vi "Flow.vi"(0 "Flow":dynamicdata(graph), 1 "Cuttoff Pressure":dbl, 5 "Interruption Time":dbl, 7 "SPL":dynamicdata(graph), 9 "File Name In":path, 11 "Error In":errorcluster, 12 "Pressure":dynamicdata(graph)) -> (2 "SPL":dbl format="%0.3f", 3 "Resistance (Out)":dbl, 4 "SGP":dbl, 6 "Interruption Time (Out)":dbl, 8 "PTP":dbl, 10 "File Name":path, 13 "Start Flow":dbl format="%0.3f", 14 "End Flow":dbl format="%0.3f", 15 "Error Out":errorcluster)   [LabVIEW 2020, in "AnalysisSupport.lvlib"]
uses:
  AnalysisSupport.lvlib
  <vilib>/Utility/miscctls.llb/LVCursorListTypeDef.ctl
  <vilib>/Analysis/baseanly.llb/Mean (DBL).vi
  <vilib>/Waveform/WDTOps.llb/WDT Get Waveform Subset DBL.vi
  <vilib>/Analysis/NI_AALBase.lvlib
panel:
  out "Derivative Flow":dynamicdata(graph)
  out "Start Time":dbl format="%#.3g"
  in  "Resistance":dbl step=5.0
  out "Subset":dynamicdata(graph)
  out "Flow":dynamicdata(graph)
  in  "Mark Flow":bool
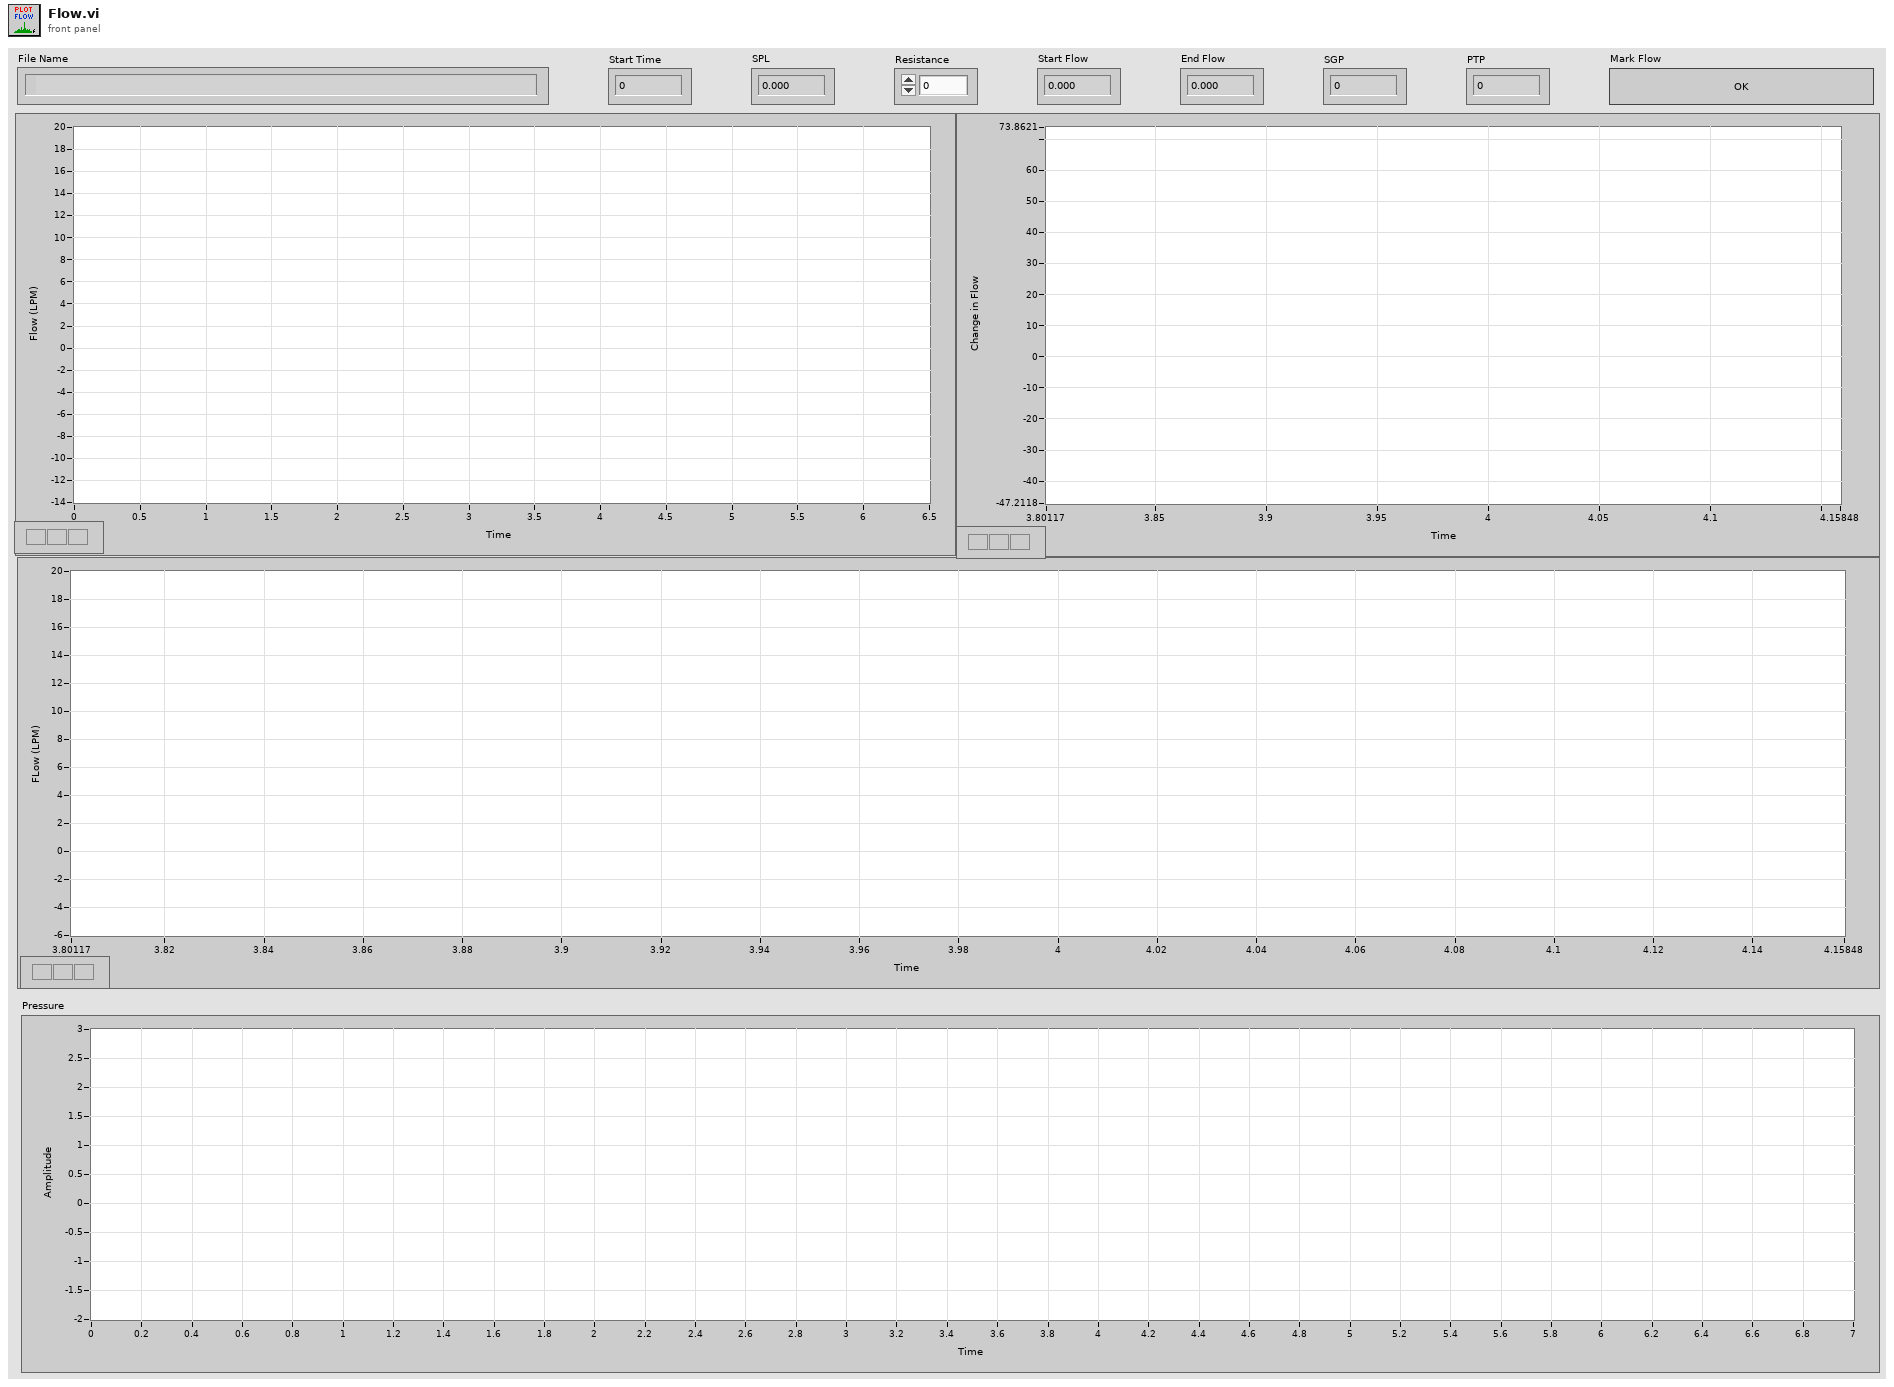
[diagram p1: front panel]
types:
  T1 = typedef "LVCursorListTypeDef.ctl" = cluster{"Name":string, "Color":u32, "Style":u8, "Point Style":u8, "Name Visible":bool, "Allow Drag":bool, "Cursor Mode":u32, "Plot":i32, "Index":i32, "Position":cluster{"X":dbl, "Y":dbl}, "X Scale":u32, "Y Scale":u32, "Watch Plots":i32[], "Watch All Plots":bool, "Plot Area":i32, "Label Offset":cluster{"X":dbl, "Y":dbl}}[]
  T2 = cluster{"Cursor List[0]":cluster{"Name":string, "Color":u32, "Style":u8, "Point Style":u8, "Name Visible":bool, "Allow Drag":bool, "Cursor Mode":u32, "Plot":i32, "Index":i32, "Position":cluster{"X":dbl, "Y":dbl}, "X Scale":u32, "Y Scale":u32, "Watch Plots":i32[], "Watch All Plots":bool, "Plot Area":i32, "Label Offset":cluster{"X":dbl, "Y":dbl}}, "Cursor List[1]":cluster{"Name":string, "Color":u32, "Style":u8, "Point Style":u8, "Name Visible":bool, "Allow Drag":bool, "Cursor Mode":u32, "Plot":i32, "Index":i32, "Position":cluster{"X":dbl, "Y":dbl}, "X Scale":u32, "Y Scale":u32, "Watch Plots":i32[], "Watch All Plots":bool, "Plot Area":i32, "Label Offset":cluster{"X":dbl, "Y":dbl}}, "Cursor List[2]":cluster{"Name":string, "Color":u32, "Style":u8, "Point Style":u8, "Name Visible":bool, "Allow Drag":bool, "Cursor Mode":u32, "Plot":i32, "Index":i32, "Position":cluster{"X":dbl, "Y":dbl}, "X Scale":u32, "Y Scale":u32, "Watch Plots":i32[], "Watch All Plots":bool, "Plot Area":i32, "Label Offset":cluster{"X":dbl, "Y":dbl}}, "Cursor List[3]":cluster{"Name":string, "Color":u32, "Style":u8, "Point Style":u8, "Name Visible":bool, "Allow Drag":bool, "Cursor Mode":u32, "Plot":i32, "Index":i32, "Position":cluster{"X":dbl, "Y":dbl}, "X Scale":u32, "Y Scale":u32, "Watch Plots":i32[], "Watch All Plots":bool, "Plot Area":i32, "Label Offset":cluster{"X":dbl, "Y":dbl}}, "Cursor List[4]":cluster{"Name":string, "Color":u32, "Style":u8, "Point Style":u8, "Name Visible":bool, "Allow Drag":bool, "Cursor Mode":u32, "Plot":i32, "Index":i32, "Position":cluster{"X":dbl, "Y":dbl}, "X Scale":u32, "Y Scale":u32, "Watch Plots":i32[], "Watch All Plots":bool, "Plot Area":i32, "Label Offset":cluster{"X":dbl, "Y":dbl}}, "Cursor List[5]":cluster{"Name":string, "Color":u32, "Style":u8, "Point Style":u8, "Name Visible":bool, "Allow Drag":bool, "Cursor Mode":u32, "Plot":i32, "Index":i32, "Position":cluster{"X":dbl, "Y":dbl}, "X Scale":u32, "Y Scale":u32, "Watch Plots":i32[], "Watch All Plots":bool, "Plot Area":i32, "Label Offset":cluster{"X":dbl, "Y":dbl}}, "Cursor List[6]":cluster{"Name":string, "Color":u32, "Style":u8, "Point Style":u8, "Name Visible":bool, "Allow Drag":bool, "Cursor Mode":u32, "Plot":i32, "Index":i32, "Position":cluster{"X":dbl, "Y":dbl}, "X Scale":u32, "Y Scale":u32, "Watch Plots":i32[], "Watch All Plots":bool, "Plot Area":i32, "Label Offset":cluster{"X":dbl, "Y":dbl}}, "Cursor List[7]":cluster{"Name":string, "Color":u32, "Style":u8, "Point Style":u8, "Name Visible":bool, "Allow Drag":bool, "Cursor Mode":u32, "Plot":i32, "Index":i32, "Position":cluster{"X":dbl, "Y":dbl}, "X Scale":u32, "Y Scale":u32, "Watch Plots":i32[], "Watch All Plots":bool, "Plot Area":i32, "Label Offset":cluster{"X":dbl, "Y":dbl}}, "Cursor List[8]":cluster{"Name":string, "Color":u32, "Style":u8, "Point Style":u8, "Name Visible":bool, "Allow Drag":bool, "Cursor Mode":u32, "Plot":i32, "Index":i32, "Position":cluster{"X":dbl, "Y":dbl}, "X Scale":u32, "Y Scale":u32, "Watch Plots":i32[], "Watch All Plots":bool, "Plot Area":i32, "Label Offset":cluster{"X":dbl, "Y":dbl}}}
  T3 = cluster{"Name":string, "Color":u32, "Style":u8, "Point Style":u8, "Name Visible":bool, "Allow Drag":bool, "Cursor Mode":u32, "Plot":i32, "Index":i32, "Position":cluster{"X":dbl, "Y":dbl}, "X Scale":u32, "Y Scale":u32, "Watch Plots":i32[], "Watch All Plots":bool, "Plot Area":i32, "Label Offset":cluster{"X":dbl, "Y":dbl}}[]
  T4 = cluster{"CrsrList[0]":cluster{"Name":string, "Color":u32, "Style":u8, "Point Style":u8, "Name Visible":bool, "Allow Drag":bool, "Cursor Mode":u32, "Plot":i32, "Index":i32, "Position":cluster{"X":dbl, "Y":dbl}, "X Scale":u32, "Y Scale":u32, "Watch Plots":i32[], "Watch All Plots":bool, "Plot Area":i32, "Label Offset":cluster{"X":dbl, "Y":dbl}}, "CrsrList[1]":cluster{"Name":string, "Color":u32, "Style":u8, "Point Style":u8, "Name Visible":bool, "Allow Drag":bool, "Cursor Mode":u32, "Plot":i32, "Index":i32, "Position":cluster{"X":dbl, "Y":dbl}, "X Scale":u32, "Y Scale":u32, "Watch Plots":i32[], "Watch All Plots":bool, "Plot Area":i32, "Label Offset":cluster{"X":dbl, "Y":dbl}}, "CrsrList[2]":cluster{"Name":string, "Color":u32, "Style":u8, "Point Style":u8, "Name Visible":bool, "Allow Drag":bool, "Cursor Mode":u32, "Plot":i32, "Index":i32, "Position":cluster{"X":dbl, "Y":dbl}, "X Scale":u32, "Y Scale":u32, "Watch Plots":i32[], "Watch All Plots":bool, "Plot Area":i32, "Label Offset":cluster{"X":dbl, "Y":dbl}}, "CrsrList[3]":cluster{"Name":string, "Color":u32, "Style":u8, "Point Style":u8, "Name Visible":bool, "Allow Drag":bool, "Cursor Mode":u32, "Plot":i32, "Index":i32, "Position":cluster{"X":dbl, "Y":dbl}, "X Scale":u32, "Y Scale":u32, "Watch Plots":i32[], "Watch All Plots":bool, "Plot Area":i32, "Label Offset":cluster{"X":dbl, "Y":dbl}}, "CrsrList[4]":cluster{"Name":string, "Color":u32, "Style":u8, "Point Style":u8, "Name Visible":bool, "Allow Drag":bool, "Cursor Mode":u32, "Plot":i32, "Index":i32, "Position":cluster{"X":dbl, "Y":dbl}, "X Scale":u32, "Y Scale":u32, "Watch Plots":i32[], "Watch All Plots":bool, "Plot Area":i32, "Label Offset":cluster{"X":dbl, "Y":dbl}}, "CrsrList[5]":cluster{"Name":string, "Color":u32, "Style":u8, "Point Style":u8, "Name Visible":bool, "Allow Drag":bool, "Cursor Mode":u32, "Plot":i32, "Index":i32, "Position":cluster{"X":dbl, "Y":dbl}, "X Scale":u32, "Y Scale":u32, "Watch Plots":i32[], "Watch All Plots":bool, "Plot Area":i32, "Label Offset":cluster{"X":dbl, "Y":dbl}}, "CrsrList[6]":cluster{"Name":string, "Color":u32, "Style":u8, "Point Style":u8, "Name Visible":bool, "Allow Drag":bool, "Cursor Mode":u32, "Plot":i32, "Index":i32, "Position":cluster{"X":dbl, "Y":dbl}, "X Scale":u32, "Y Scale":u32, "Watch Plots":i32[], "Watch All Plots":bool, "Plot Area":i32, "Label Offset":cluster{"X":dbl, "Y":dbl}}, "CrsrList[7]":cluster{"Name":string, "Color":u32, "Style":u8, "Point Style":u8, "Name Visible":bool, "Allow Drag":bool, "Cursor Mode":u32, "Plot":i32, "Index":i32, "Position":cluster{"X":dbl, "Y":dbl}, "X Scale":u32, "Y Scale":u32, "Watch Plots":i32[], "Watch All Plots":bool, "Plot Area":i32, "Label Offset":cluster{"X":dbl, "Y":dbl}}, "CrsrList[8]":cluster{"Name":string, "Color":u32, "Style":u8, "Point Style":u8, "Name Visible":bool, "Allow Drag":bool, "Cursor Mode":u32, "Plot":i32, "Index":i32, "Position":cluster{"X":dbl, "Y":dbl}, "X Scale":u32, "Y Scale":u32, "Watch Plots":i32[], "Watch All Plots":bool, "Plot Area":i32, "Label Offset":cluster{"X":dbl, "Y":dbl}}}
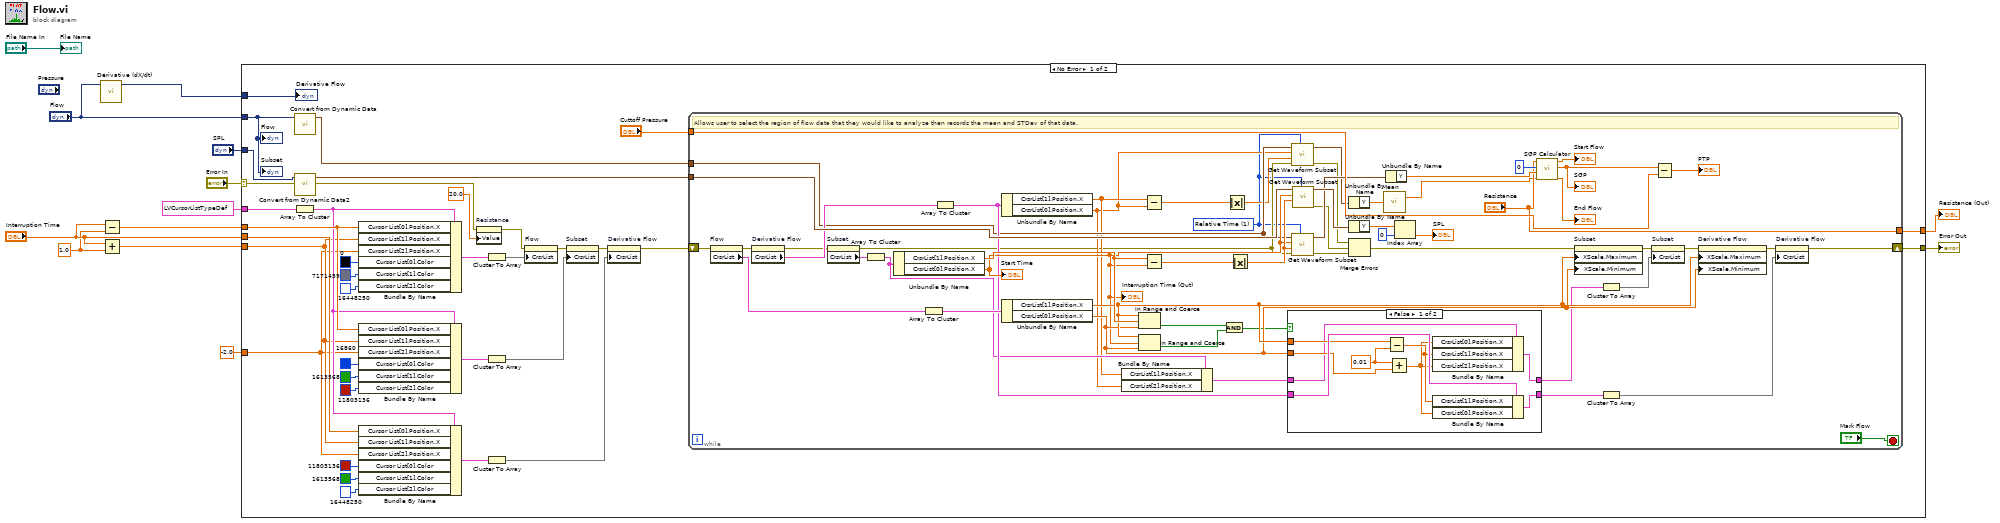
[diagram p0: block diagram]
diagram:
  w3 = 1.0 ("y")
  n1 = call "Derivative (dX/dt)"("Signals"="Flow") -> ("Result"=w5:dynamicdata)  [unwired: 5 in, 1 out]
  n2 = Subtract(x="Interruption Time", y=w3) -> (x-y=w7:dbl)
  n3 = Add(x="Interruption Time", y=w3) -> (x+y=w4:dbl)
  n4 = case shown="No Error" "Error In" {
    selector: "Error In" -> [w29 w116]
    tunnel: "Flow" -> [w47 _]
    tunnel: [w48 w116] -> w11
    tunnel: "Interruption Time" -> [w44 _]
    tunnel: T1 [{"Name"="Left", "Color"=9843450, "Style"=2, "Point Style"=1, "Name Visible"=FALSE, "Allow Drag"=TRUE, "Cursor Mode"=0, "Plot"=0, "Index"=0, "Position"={"X"=3.0, "Y"=0.0}, "X Scale"=0, "Y Scale"=0, "Watch Plots"=[], "Watch All Plots"=FALSE, "Plot Area"=0, "Label Offset"={"X"=0.0, "Y"=0.0}}, {"Name"="Right", "Color"=681210, "Style"=2, "Point Style"=1, "Name Visible"=FALSE, "Allow Drag"=TRUE, "Cursor Mode"=0, "Plot"=0, "Index"=0, "Position"={"X"=3.5, "Y"=0.0}, "X Scale"=0, "Y Scale"=0, "Watch Plots"=[], "Watch All Plots"=FALSE, "Plot Area"=0, "Label Offset"={"X"=0.0, "Y"=0.0}}, {"Name"="Middle", "Color"=4617539, "Style"=2, "Point Style"=1, "Name Visible"=FALSE, "Allow Drag"=TRUE, "Cursor Mode"=0, "Plot"=0, "Index"=0, "Position"={"X"=0.0, "Y"=0.0}, "X Scale"=0, "Y Scale"=0, "Watch Plots"=[], "Watch All Plots"=FALSE, "Plot Area"=0, "Label Offset"={"X"=0.0, "Y"=0.0}}] ("Cursor List") -> [w45 _]
    tunnel: [w42 _] -> w9
    tunnel: w4 -> [w24 _]
    tunnel: w7 -> [w26 _]
    tunnel: "SPL" -> [w37 _]
    tunnel: w5 -> [w34 _]
    tunnel: -2.0 -> [w23 _]
    frame No Error {
      n5 = call "Convert from Dynamic Data"("Dynamic Data Type"=w47) -> ("Waveform"=w46:waveform(dbl))  [unwired: 3 in]
      n6 = call "Convert from Dynamic Data2"("Dynamic Data Type"=w37) -> ("Waveform"=w36:waveform(dbl))  [unwired: 3 in]
      n7 = Array To Cluster(array=w45) -> (cluster=w25:T2)
      n8 = Bundle By Name(cluster=w25, "Cursor List[0].Position.X"=w26, "Cursor List[1].Position.X"=w24, "Cursor List[2].Position.X"=w23, "Cursor List[0].Color"=u32 0, "Cursor List[1].Color"=u32 7171459, "Cursor List[2].Color"=u32 16448250) -> (w40:T2)
      n9 = Bundle By Name(cluster=w25, "Cursor List[0].Position.X"=w26, "Cursor List[1].Position.X"=w24, "Cursor List[2].Position.X"=w23, "Cursor List[0].Color"=u32 16860, "Cursor List[1].Color"=u32 1613568, "Cursor List[2].Color"=u32 11803136) -> (w28:T2)
      n10 = Bundle By Name(cluster=w25, "Cursor List[0].Position.X"=w44, "Cursor List[1].Position.X"=w24, "Cursor List[2].Position.X"=w23, "Cursor List[0].Color"=u32 11803136, "Cursor List[1].Color"=u32 1613568, "Cursor List[2].Color"=u32 16448250) -> (w43:T2)
      n11 = property on="Resistance" class="DigNum (strict)"(error in=w29, "Value"=20.0 ("Resistance")) -> (error out=w30:errorcluster)  [unwired: 1 in, 1 out]
      n12 = Cluster To Array(cluster=w40) -> (array=w39:T3)
      n13 = Cluster To Array(cluster=w28) -> (array=w27:T3)
      n14 = Cluster To Array(cluster=w43) -> (array=w31:T3)
      n15 = property on="Flow" class="WFGraph (strict)"(error in=w30, "CrsrList"=w39) -> (error out=w41:errorcluster)  [unwired: 1 in, 1 out]
      n16 = property on="Subset" class="WFGraph (strict)"(error in=w41, "CrsrList"=w27) -> (error out=w33:errorcluster)  [unwired: 1 in, 1 out]
      n17 = property on="Derivative Flow" class="WFGraph (strict)"(error in=w33, "CrsrList"=w31) -> (error out=w32:errorcluster)  [unwired: 1 in, 1 out]
      n18 = while {
        shift-right: [w71] -> w48
        shift-left: w32 -> [w77]
        tunnel: w46 -> [w68]
        tunnel: ["Resistance"] -> w42
        tunnel: w36 -> [w97]
        tunnel: "Cuttoff Pressure" -> [w96]
        stop <- "Mark Flow" stop-if-true
        w49 = u16 1 items=["Samples", "Relative Time"] ("start/duration format")
        # "Allows user to select the region of flow data that they would like to analyze then records the mean and STDev of that data."
        n19 = property on="Flow" class="WFGraph (strict)"(error in=w77) -> (error out=w55:errorcluster, "CrsrList"=w102:T1)  [unwired: 1 in, 1 out]
        n20 = property on="Derivative Flow" class="WFGraph (strict)"(error in=w55) -> (error out=w54:errorcluster, "CrsrList"=w95:T1)  [unwired: 1 in, 1 out]
        n21 = property on="Subset" class="WFGraph (strict)"(error in=w54) -> (error out=w52:errorcluster, "CrsrList"=w101:T1)  [unwired: 1 in, 1 out]
        n22 = Array To Cluster(array=w101) -> (cluster=w67:T4)
        n23 = Unbundle By Name(w67) -> ("CrsrList[1].Position.X"=w100:dbl, "CrsrList[0].Position.X"=w78:dbl)
        "Interruption Time (Out)" <- w78
        "Start Time" <- w78
        n24 = Array To Cluster(array=w102) -> (cluster=w103:T4)
        n25 = Array To Cluster(array=w95) -> (cluster=w70:T4)
        n26 = Unbundle By Name(w70) -> ("CrsrList[1].Position.X"=w59:dbl, "CrsrList[0].Position.X"=w58:dbl)
        n27 = Unbundle By Name(w103) -> ("CrsrList[1].Position.X"=w99:dbl, "CrsrList[0].Position.X"=w98:dbl)
        n28 = Bundle By Name(cluster=w67, "CrsrList[1].Position.X"=w59, "CrsrList[2].Position.X"=w58) -> (w66:T4)
        n29 = In Range and Coerce(upper limit=w99, x=w100, lower limit=w98) -> (In Range?=w93:bool)  [unwired: 1 out]
        n30 = In Range and Coerce(upper limit=w99, x=w78, lower limit=w98) -> (In Range?=w92:bool)  [unwired: 1 out]
        n31 = Subtract(x=w59, y=w58) -> (x-y=w60:dbl)
        n32 = Subtract(x=w100, y=w78) -> (x-y=w90:dbl)
        n33 = And(x=w93, y=w92) -> (x .and. y?=w91:bool)
        n34 = Absolute Value(x=w60) -> (abs(x)=w61:dbl)
        n35 = Absolute Value(x=w90) -> (abs(x)=w86:dbl)
        n36 = case shown="False" w91 {
          tunnel: w70 -> [w113 w115]
          tunnel: [w112 w115] -> w94
          tunnel: w99 -> [w111 _]
          tunnel: w98 -> [w110 _]
          tunnel: w66 -> [w109 w114]
          tunnel: [w108 w114] -> w74
          frame False {
            w107 = 0.01 ("y")
            # "Right Cursor"
            n37 = Subtract(x=w111, y=w107) -> (x-y=w106:dbl)
            n38 = Add(x=w107, y=w110) -> (x+y=w105:dbl)
            n39 = Bundle By Name(cluster=w109, "CrsrList[0].Position.X"=w105, "CrsrList[1].Position.X"=w106, "CrsrList[2].Position.X"=w105) -> (w108:T4)
            n40 = Bundle By Name(cluster=w113, "CrsrList[1].Position.X"=w106, "CrsrList[0].Position.X"=w105) -> (w112:T4)
          }
          frame True {
            # "Right Cursor"
          }
        }
        n41 = call-poly <vilib>:"Get Waveform Subset.vi"("start/duration format"=w49, "error in (no error)"=w52, "duration"=w61, "start samples/time"=w58, "waveform in"=w68) -> ("error out"=w57:errorcluster, "waveform out"=w64:waveform(dbl))  [unwired: 1 in, 2 out]
        n42 = call-poly <vilib>:"Get Waveform Subset.vi"("start/duration format"=w49, "error in (no error)"=w52, "duration"=w86, "start samples/time"=w78, "waveform in"=w68) -> ("error out"=w50:errorcluster, "waveform out"=w69:waveform(dbl))  [unwired: 1 in, 2 out]
        n43 = call-poly <vilib>:"Get Waveform Subset.vi"("start/duration format"=w49, "duration"=w86, "start samples/time"=w78, "waveform in"=w97) -> ("error out"=w56:errorcluster, "waveform out"=w87:waveform(dbl))  [unwired: 2 in, 2 out]
        n44 = Unbundle By Name(w64) -> ("Y"=w63:dbl[])
        n45 = Unbundle By Name(w87) -> ("Y"=w85:dbl[])
        n46 = Merge Errors(w57, w56, w50) -> (w51:errorcluster)
        n47 = call-poly <vilib>:"Mean.vi"("X"=w63) -> ("mean"=w62:dbl)  [unwired: 1 out]
        n48 = Unbundle By Name(w69) -> ("Y"=w88:dbl[])
        n49 = Index Array(array=w85, index=0 ("Start Index")) -> (element=→"SPL":dbl)
        n50 = call "SGP Calculator.vi"("End Flow"=w62, "Flow Array"=w88, "Start Index"=0, "Resistance"="Resistance") -> ("End Flow Out"=→"End Flow":dbl, "SGP"=w80:dbl, "Start Flow"=→"Start Flow":dbl)  [unwired: 5 in]
        "SGP" <- w80
        n51 = property on="Subset" class="WFGraph (strict)"(error in=w51, "XScale.Maximum"=w99, "XScale.Minimum"=w98) -> (error out=w76:errorcluster)  [unwired: 1 in, 1 out]
        n52 = Cluster To Array(cluster=w74) -> (array=w73:T3)
        n53 = Cluster To Array(cluster=w94) -> (array=w75:T3)
        n54 = property on="Subset" class="WFGraph (strict)"(error in=w76, "CrsrList"=w73) -> (error out=w53:errorcluster)  [unwired: 1 in, 1 out]
        n55 = Subtract(x=w80, y=w96) -> (x-y=→"PTP":dbl)
        n56 = property on="Derivative Flow" class="WFGraph (strict)"(error in=w53, "XScale.Maximum"=w99, "XScale.Minimum"=w98) -> (error out=w72:errorcluster)  [unwired: 1 in, 1 out]
        n57 = property on="Derivative Flow" class="WFGraph (strict)"(error in=w72, "CrsrList"=w75) -> (error out=w71:errorcluster)  [unwired: 1 in, 1 out]
      }
      "Flow" <- w47
      "Subset" <- w47
      "Derivative Flow" <- w34
    }
    frame Error {
    }
  }
  "Error Out" <- w11
  "Resistance (Out)" <- w9
  "File Name" <- "File Name In"
